vi "FTW-Scheduler-GetNextJob.vi"(0 "FTW Job Scheduler":refnum<class "FTW-Scheduler.lvclass">, 7 "Jobs Performed":i32, 11 "error in":errorcluster) -> (4 "FTW Job Scheduler out":refnum<class "FTW-Scheduler.lvclass">, 6 "Time til Next Scheduled Job":i32=20 format="%d msec", 8 "Current Job":string, 15 "error out":errorcluster)   [LabVIEW 2015, in "FTW-Scheduler.lvclass"]
uses:
  FTW-Scheduler.lvclass
  job/FTW-ScheduledJob.lvclass
panel:
  # "Inputs"
  # "Outputs"
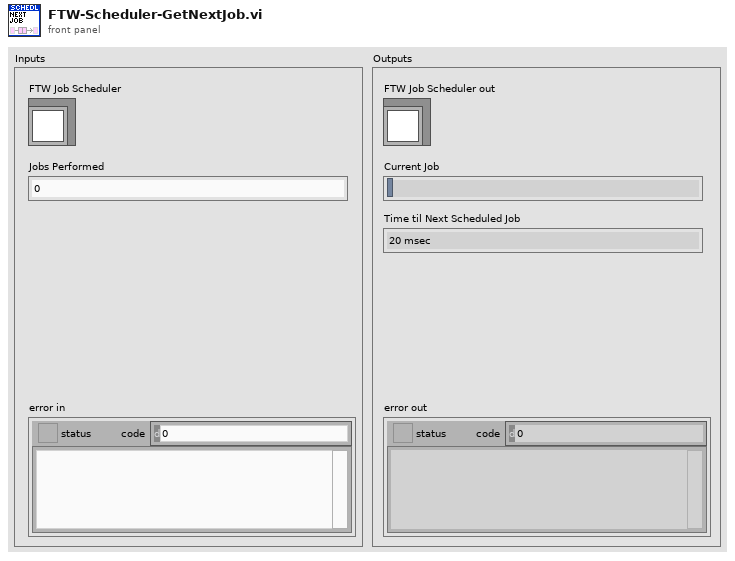
[diagram p1: front panel]
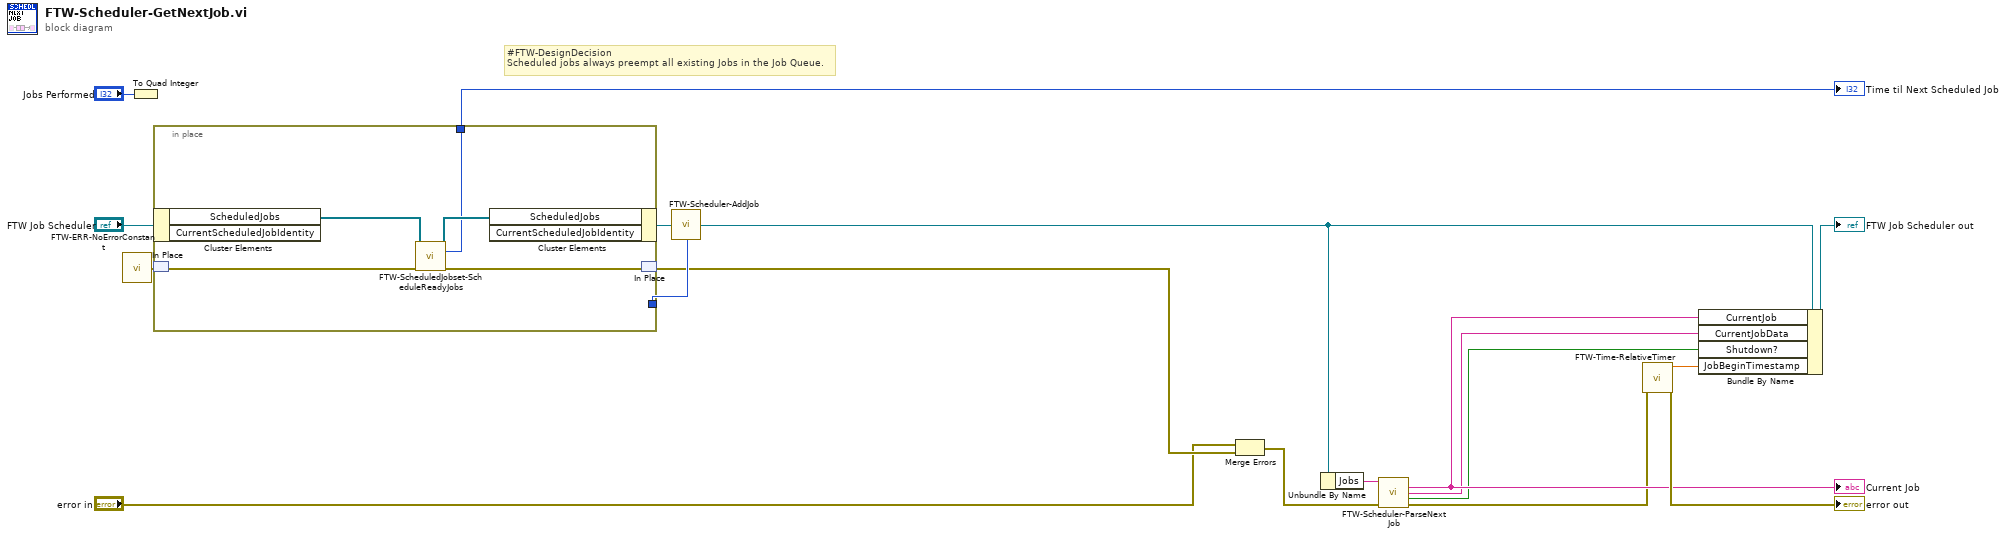
[diagram p0: block diagram]
diagram:
  # "#FTW-DesignDecision\nScheduled jobs always preempt all existing Jobs in the Job Queue."
  n1 = call "FTW-ERR-NoErrorConstant.vi"() -> ("no error"=w10:errorcluster)
  n2 = To Quad Integer(1:"Jobs Performed") -> ()  [unwired: 1 out]
  n3 = in-place {
    in-place-border: [w21] -> w15
    in-place-border: [_] -> w13
    n4 = in-place-cluster #1("FTW Job Scheduler") -> ("ScheduledJobs"=w22:refnum<class "FTW-ScheduledJob.lvclass">[], "CurrentScheduledJobIdentity"=w20:string)
    n5 = in-place-match #2(w10) -> (w24:errorcluster)
    n6 = call "FTW-ScheduledJobset-ScheduleReadyJobs.vi"("FTW Scheduled Jobset"=w22, "error in"=w24) -> ("FTW Scheduled Jobset out"=w25:refnum<class "FTW-ScheduledJob.lvclass">[], "Scheduled Job Index to Run Now"=w21:i32, "error out"=w23:errorcluster)  [unwired: 10 in, 1 out]
    n7 = in-place-cluster #1("ScheduledJobs"=w25) -> (w14:refnum<class "FTW-Scheduler.lvclass">)  [unwired: 1 in]
    n8 = in-place-match #2(w23) -> (w3:errorcluster)
  }
  "Time til Next Scheduled Job" <- w15
  n9 = call "FTW-Scheduler-AddJob.vi"("Add to Job Sequence"=w13, "FTW Job Scheduler"=w14) -> ("FTW Job Scheduler out"=w6:refnum<class "FTW-Scheduler.lvclass">)  [unwired: 2 in]
  n10 = Merge Errors("error in", w3) -> (w1:errorcluster)
  n11 = Unbundle By Name(w6) -> ("Jobs"=w9:string)
  n12 = call "FTW-Scheduler-ParseNextJob.vi"("Jobs"=w9, "error in"=w1) -> ("Jobs out"=w7:string, "CurrentJob"=w12:string, "CurrentJobData"=w11:string, "Shutdown?"=w8:bool, "error out"=w5:errorcluster)  [unwired: 9 in]
  "Current Job" <- w12
  n13 = call "FTW-Time-RelativeTimer.vi"("error in"=w5) -> ("Current Timer Value"=w4:dbl, "error out"=→"error out":errorcluster)  [unwired: 12 in, 1 out]
  n14 = Bundle By Name(cluster=w6, "CurrentJob"=w12, "CurrentJobData"=w11, "Shutdown?"=w8, "JobBeginTimestamp"=w4) -> (→"FTW Job Scheduler out":refnum<class "FTW-Scheduler.lvclass">)
